vi "Background_Binned.vi"(11 "Background Array":dbl[][](array[numeric])) -> (0 "Binned Array 10":dbl[][](array[numeric]), 1 "Binned Array 4":dbl[][](array[numeric]), 2 "Binned Array 2":dbl[][](array[numeric]), 3 "Binned Array 1":dbl[][](array[numeric]))   [LabVIEW 2013]
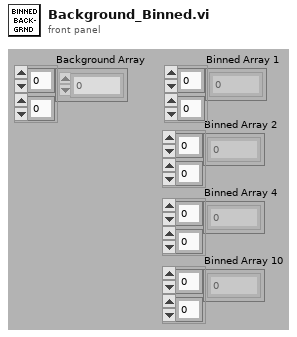
[diagram p1: front panel]
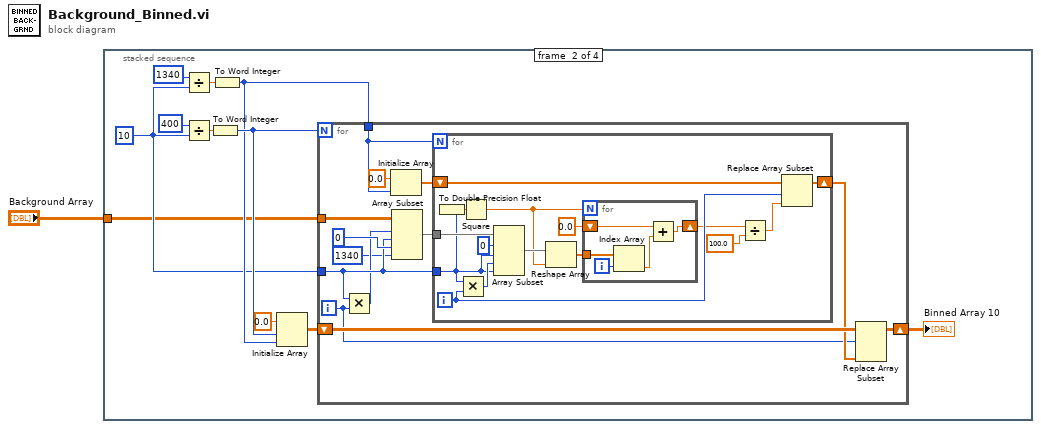
[diagram p0: block diagram]
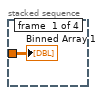
[diagram p2: hidden frame]
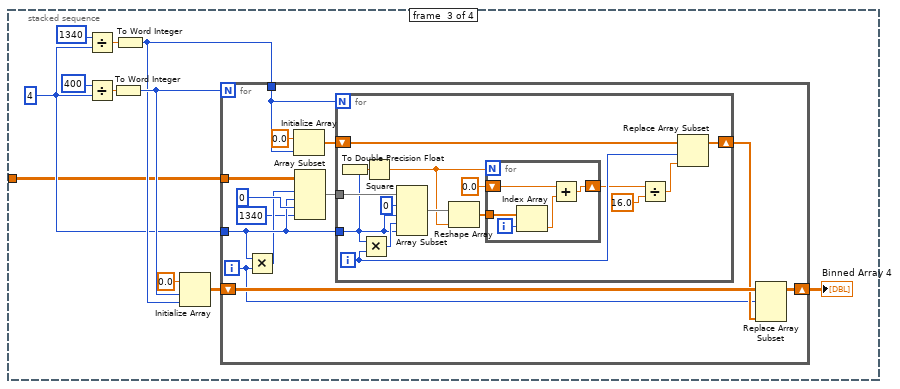
[diagram p3: hidden frame]
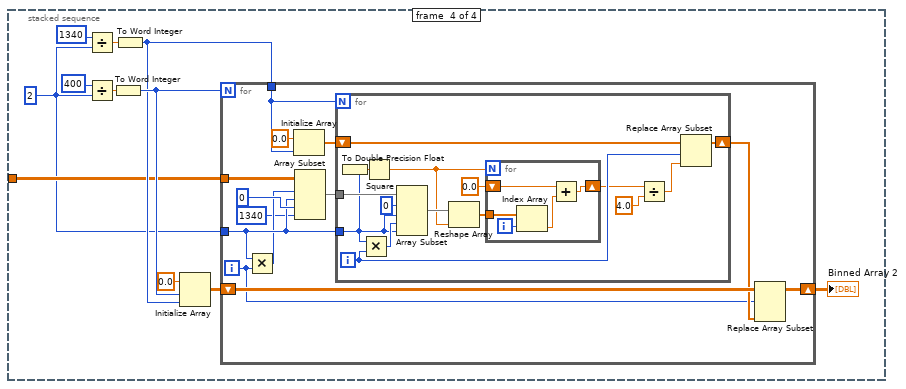
[diagram p4: hidden frame]
diagram:
  n1 = stacked-sequence {
    tunnel: "Background Array" -> [w2 w3 w47 w92]
    frame #0 {
      "Binned Array 1" <- w2
    }
    frame #1 {
      w4 = u32 10 ("Binning")
      n2 = Divide(x=u32 1340, y=w4) -> (x/y=w11:dbl)
      n3 = Divide(x=u32 400, y=w4) -> (x/y=w10:dbl)
      n4 = To Word Integer(number=w10) -> (16bit integer=w8:i16)
      n5 = To Word Integer(number=w11) -> (16bit integer=w7:i16)
      n6 = Initialize Array(0.0 ("element"), w8, w7) -> (w6:dbl[][])
      n7 = for {
        N: w8 -> [_]
        tunnel: w7 -> [w18]
        tunnel: w4 -> [w16]
        shift-right: [w22] -> w5
        shift-left: w6 -> [w23]
        tunnel: w3 -> [w26]
        i -> [w17]
        n8 = Multiply(x=w16, y=w17) -> (x*y=w15:u32)
        n9 = Initialize Array(0.0 ("element"), w18) -> (w19:dbl[])
        n10 = Array Subset(array=w26, index (row)=w15, length (row)=w16, index (col)=0 ("index"), length (col)=1340 ("length")) -> (w25:dbl[][])
        n11 = for {
          N: w18 -> [_]
          tunnel: w16 -> [w34]
          tunnel: w25 -> [w41]
          shift-right: [w39] -> w21
          shift-left: w19 -> [w38]
          i -> [w37]
          n12 = To Double Precision Float(number=w34) -> (double precision float=w27:dbl)
          n13 = Multiply(x=w34, y=w37) -> (x*y=w36:u32)
          n14 = Square(x=w27) -> (x^2=w31:dbl)
          n15 = Array Subset(array=w41, index (row)=0 ("index"), length (row)=w34, index (col)=w36, length (col)=w34) -> (w35:dbl[][])
          n16 = Reshape Array(w35, w31) -> (w33:dbl[])
          n17 = for {
            N: w31 -> [_]
            tunnel: w33 -> [w46]
            shift-right: [w43] -> w30
            shift-left: 0.0 -> [w42]
            i -> [w45]
            n18 = Index Array(array=w46, index=w45) -> (element=w44:dbl)
            n19 = Add(x=w42, y=w44) -> (x+y=w43:dbl)
          }
          n20 = Divide(x=w30, y=100.0) -> (x/y=w29:dbl)
          n21 = Replace Array Subset(array=w38, new element=w29, index=w37) -> (w39:dbl[])
        }
        n22 = Replace Array Subset(array=w23, new element=w21, index (row)=w17) -> (w22:dbl[][])  [unwired: 1 in]
      }
      "Binned Array 10" <- w5
    }
    frame #2 {
      w48 = u32 4 ("Binning")
      n23 = Divide(x=u32 1340, y=w48) -> (x/y=w55:dbl)
      n24 = Divide(x=u32 400, y=w48) -> (x/y=w54:dbl)
      n25 = To Word Integer(number=w54) -> (16bit integer=w52:i16)
      n26 = To Word Integer(number=w55) -> (16bit integer=w51:i16)
      n27 = Initialize Array(0.0 ("element"), w52, w51) -> (w50:dbl[][])
      n28 = for {
        N: w52 -> [_]
        tunnel: w51 -> [w62]
        tunnel: w48 -> [w60]
        shift-right: [w66] -> w49
        shift-left: w50 -> [w67]
        tunnel: w47 -> [w70]
        i -> [w61]
        n29 = Multiply(x=w60, y=w61) -> (x*y=w59:u32)
        n30 = Initialize Array(0.0 ("element"), w62) -> (w63:dbl[])
        n31 = Array Subset(array=w70, index (row)=w59, length (row)=w60, index (col)=0 ("index"), length (col)=1340 ("length")) -> (w69:dbl[][])
        n32 = for {
          N: w62 -> [_]
          tunnel: w60 -> [w78]
          tunnel: w69 -> [w85]
          shift-right: [w83] -> w65
          shift-left: w63 -> [w82]
          i -> [w81]
          n33 = To Double Precision Float(number=w78) -> (double precision float=w71:dbl)
          n34 = Multiply(x=w78, y=w81) -> (x*y=w80:u32)
          n35 = Square(x=w71) -> (x^2=w75:dbl)
          n36 = Array Subset(array=w85, index (row)=0 ("index"), length (row)=w78, index (col)=w80, length (col)=w78) -> (w79:dbl[][])
          n37 = Reshape Array(w79, w75) -> (w77:dbl[])
          n38 = for {
            N: w75 -> [_]
            tunnel: w77 -> [w90]
            shift-right: [w87] -> w74
            shift-left: 0.0 -> [w86]
            i -> [w89]
            n39 = Index Array(array=w90, index=w89) -> (element=w88:dbl)
            n40 = Add(x=w86, y=w88) -> (x+y=w87:dbl)
          }
          n41 = Divide(x=w74, y=16.0) -> (x/y=w73:dbl)
          n42 = Replace Array Subset(array=w82, new element=w73, index=w81) -> (w83:dbl[])
        }
        n43 = Replace Array Subset(array=w67, new element=w65, index (row)=w61) -> (w66:dbl[][])  [unwired: 1 in]
      }
      "Binned Array 4" <- w49
    }
    frame #3 {
      w91 = u32 2 ("Binning")
      n44 = Divide(x=u32 1340, y=w91) -> (x/y=w99:dbl)
      n45 = Divide(x=u32 400, y=w91) -> (x/y=w98:dbl)
      n46 = To Word Integer(number=w98) -> (16bit integer=w96:i16)
      n47 = To Word Integer(number=w99) -> (16bit integer=w95:i16)
      n48 = Initialize Array(0.0 ("element"), w96, w95) -> (w94:dbl[][])
      n49 = for {
        N: w96 -> [_]
        tunnel: w95 -> [w106]
        tunnel: w91 -> [w104]
        shift-right: [w110] -> w93
        shift-left: w94 -> [w111]
        tunnel: w92 -> [w114]
        i -> [w105]
        n50 = Multiply(x=w104, y=w105) -> (x*y=w103:u32)
        n51 = Initialize Array(0.0 ("element"), w106) -> (w107:dbl[])
        n52 = Array Subset(array=w114, index (row)=w103, length (row)=w104, index (col)=0 ("index"), length (col)=1340 ("length")) -> (w113:dbl[][])
        n53 = for {
          N: w106 -> [_]
          tunnel: w104 -> [w122]
          tunnel: w113 -> [w129]
          shift-right: [w127] -> w109
          shift-left: w107 -> [w126]
          i -> [w125]
          n54 = To Double Precision Float(number=w122) -> (double precision float=w115:dbl)
          n55 = Multiply(x=w122, y=w125) -> (x*y=w124:u32)
          n56 = Square(x=w115) -> (x^2=w119:dbl)
          n57 = Array Subset(array=w129, index (row)=0 ("index"), length (row)=w122, index (col)=w124, length (col)=w122) -> (w123:dbl[][])
          n58 = Reshape Array(w123, w119) -> (w121:dbl[])
          n59 = for {
            N: w119 -> [_]
            tunnel: w121 -> [w134]
            shift-right: [w131] -> w118
            shift-left: 0.0 -> [w130]
            i -> [w133]
            n60 = Index Array(array=w134, index=w133) -> (element=w132:dbl)
            n61 = Add(x=w130, y=w132) -> (x+y=w131:dbl)
          }
          n62 = Divide(x=w118, y=4.0) -> (x/y=w116:dbl)
          n63 = Replace Array Subset(array=w126, new element=w116, index=w125) -> (w127:dbl[])
        }
        n64 = Replace Array Subset(array=w111, new element=w109, index (row)=w105) -> (w110:dbl[][])  [unwired: 1 in]
      }
      "Binned Array 2" <- w93
    }
  }
